vi "HelioView.vi"() -> ()   [LabVIEW 2010]
uses:
  common/xcontrols/XImage/XImage/XImage.xctl
  common/classes/ImageCollection/ImageCollection/ImageCollection.lvclass
panel:
  in  "XImage":refnum<class "ImageCollection.lvclass">(xcontrol)
  in  "stopBtn":bool
  out "error out":errorcluster
  in  "error in (no error)":errorcluster
  # "HelioView"
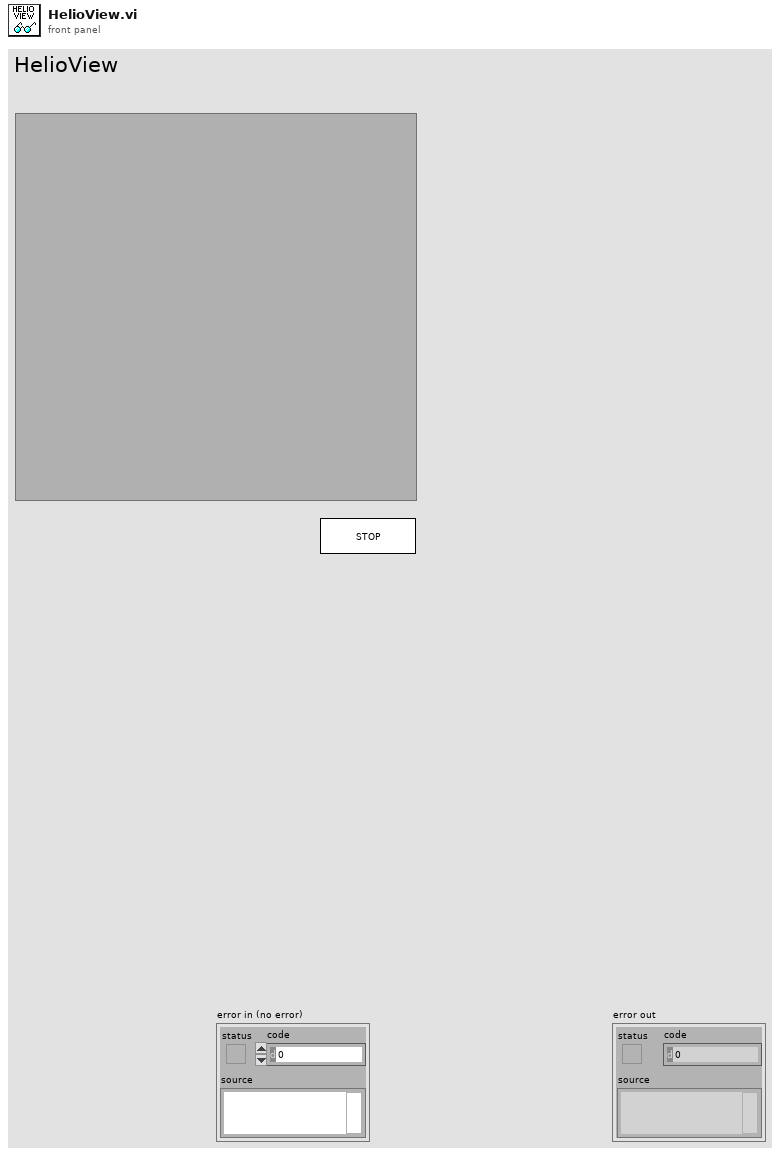
[diagram p1: front panel]
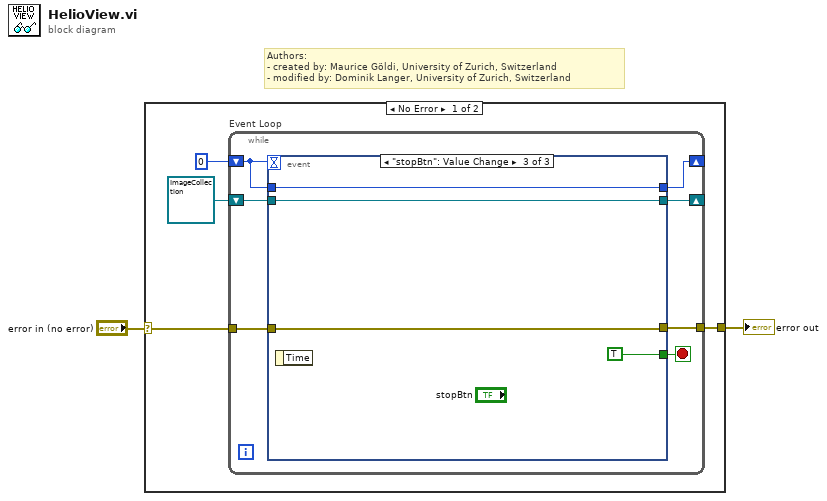
[diagram p0: block diagram]
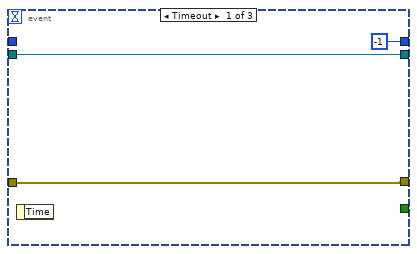
[diagram p2: hidden frame]
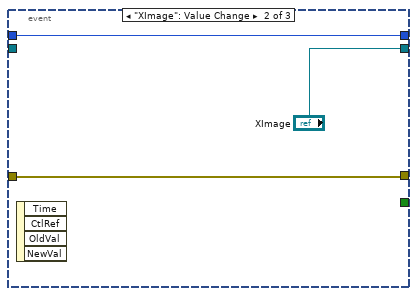
[diagram p3: hidden frame]
diagram:
  # "Authors: \n- created by: Maurice Göldi, University of Zurich, Switzerland\n- modified by: Dominik Langer, University of Zurich, Switzerland"
  n1 = case shown="No Error" "error in (no error)" {
    selector: "error in (no error)" -> [w5 w24]
    tunnel: [w4 w24] -> w1
    frame No Error {
      n2 = while "Event Loop" {
        shift-right: [w12] -> _
        shift-left: 0 -> [w13]
        tunnel: w5 -> [w11]
        tunnel: [w10] -> w4
        shift-right: [w7] -> _
        shift-left: refnum<class "ImageCollection.lvclass"> refnum ("XImage") -> [w9]
        stop <- w8 stop-if-true
        n3 = event shown="[2] \"stopBtn\": Value Change" {
          selector: _ -> [_ _ _]
          dyn-events: _ -> [_ _ _]
          timeout: w13 -> [_ _ _]
          tunnel: w13 -> [_ w19 w23]
          tunnel: [-1 w19 w23] -> w12
          tunnel: [w15 w18 w21] -> w10
          tunnel: w11 -> [w15 w18 w21]
          tunnel: w9 -> [w14 _ w20]
          tunnel: [_ _ TRUE] -> w8
          tunnel: [w14 "XImage" w20] -> w7
          event Timeout {
            n4 = event-data() -> ()  [unwired: 1 in, 1 out]
          }
          event "XImage": Value Change {
            n5 = event-data() -> ()  [unwired: 1 in, 4 out]
          }
          event "stopBtn": Value Change {
            n6 = event-data() -> ()  [unwired: 1 in, 1 out]
          }
        }
      }
    }
    frame Error {
    }
  }
  "error out" <- w1
